vi "Initialization Globals.vi"() -> ()   [LabVIEW 2019]
uses:
  Enum_FileNewInterval.ctl
panel:
  out "Watchdog Enable":bool
  in  "Stbd 3 Phase Current Scaling":dbl[](array[numeric])=[-12.724, -12.739, -12.73]
  in  "Stbd 3 Phase Voltage Scaling":dbl[](array[numeric])=[50.0, 50.0, 50.0]
  out "AWS Enable Upload (TDMS)":bool
  in  "Scaling Factors Grp0":dbl[](array[numeric])
  in  "PowGrp0 samples per channel":i32=2500
  in  "PowGrp0 sample rate [Hz]":dbl=5000.0 format="%0.2f"
  out "Save Raw Data (3ph only)":bool=TRUE
  out "Raw Interval Time Remaining":dbl format="%<%H:%M:%S%1u>t"
  out "Raw Sampling Time Remaining":dbl format="%<%H:%M:%S%1u>t"
  out "Save Raw Data":bool=TRUE
  out "Raw Data Mode":string="Continuous"
  out "Raw Sampling Time (min)":i32=120
  out "Raw Interval (min)":i32=600
  in  "Data Folder Path":string
  in  "Config File Path":string
  out "AWS Enable Upload (Summary)":bool=TRUE
  in  "AWS Bucket":string
  in  "AWS Secret Key":string
  in  "AWS Access Key":string
  out "Summary Upload Interval pow (min)":i32=10
  in  "Local file path (pow)":string
  in  "Destination write path (pow)":string
  in  "File Write Interval":T1
  out "CSV Loop Delay (ms)":i32=500
  out "CSV Avg Time (Sec)":i32=600
  out "Enable CSV Summary File?":bool=TRUE
  out "Summary Upload Interval pos (min)":i32=10
  out "FTP Delete After Upload?":bool
  out "Enable FTP?":bool
  in  "Destination write path (pos)":string
  in  "Local file path (pos)":string
  in  "FTP Password":string
  in  "FTP User":string
  in  "FTP Host":string
  out "Send Alert Email":bool
  out "Email Password":string="wqrguvwsznpmzczp"
  out "Email Username":string="nrel.daq@gmail.com"
  out "Outgoing SMTP":string="smtp.gmail.com"
  out "Sender Email":string="nrel.daq@gmail.com"
  out "Email DL 1":string="robert.raye@nrel.gov"
  out "Email DL 2":string="robert.raye@nrel.gov,casey.nichols@nrel.gov,lrummel@cpower.co,jprudell@cpower.co,mark.murphy@nrel.gov"
  out "Enable Email Alerts?":bool
  out "AWOL Snooze":dbl=15.0
  out "Red Snooze":dbl=60.0
  out "Yellow Snooze":dbl=60.0
  out "AWOL Radius":dbl=5.0
  out "Red Radius":dbl=2.5
  out "Yellow Radius":dbl=2.0
  out "Set Point Lon":dbl=-105.228346
  out "Set Point Lat":dbl=39.9132
  out "Watchdog Period":u32=2000
  out "Reset target on WD TO":bool
  # "I/O Configs"
  # "Watch Circle"
  # "Files and Uploads"
  # "PT-EN0-1001"
  # "PT-EN0-1002"
  # "PT-EN0-1003"
  # "CT-EN0-1001"
  # "CT-EN0-1002"
  # "CT-EN0-1003"
  # "Watchdog Timer"
  # "Not Used/Remove from Configurator"
  # "Control Setpoints and Thresholds"
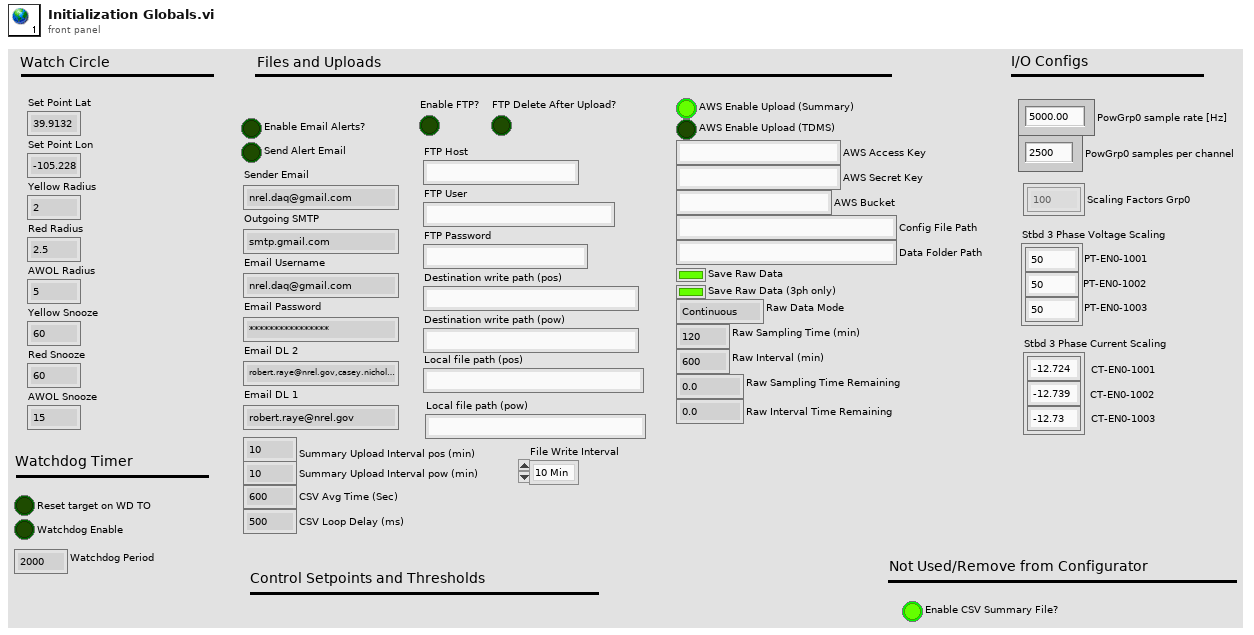
[diagram p1: front panel]
types:
  T1 = typedef "Enum_FileNewInterval.ctl" = enum16{"10 Min", "Hourly", "Daily", "Weekly", "Monthly"}
diagram:
